vi "Merge Array.vi"(8 "Start array":i32, 9 "prev index":i32, 11 "array":T1) -> (3 "array out":T1)   [LabVIEW 2014]
uses:
  Libraries/Map Data Folder/All-Lines.ctl
  Libraries/Map Data Folder/LineCluster.ctl
  Libraries/Map Data Folder/LineConnection.ctl
  Libraries/Map Data Folder/Map Data.lvlib
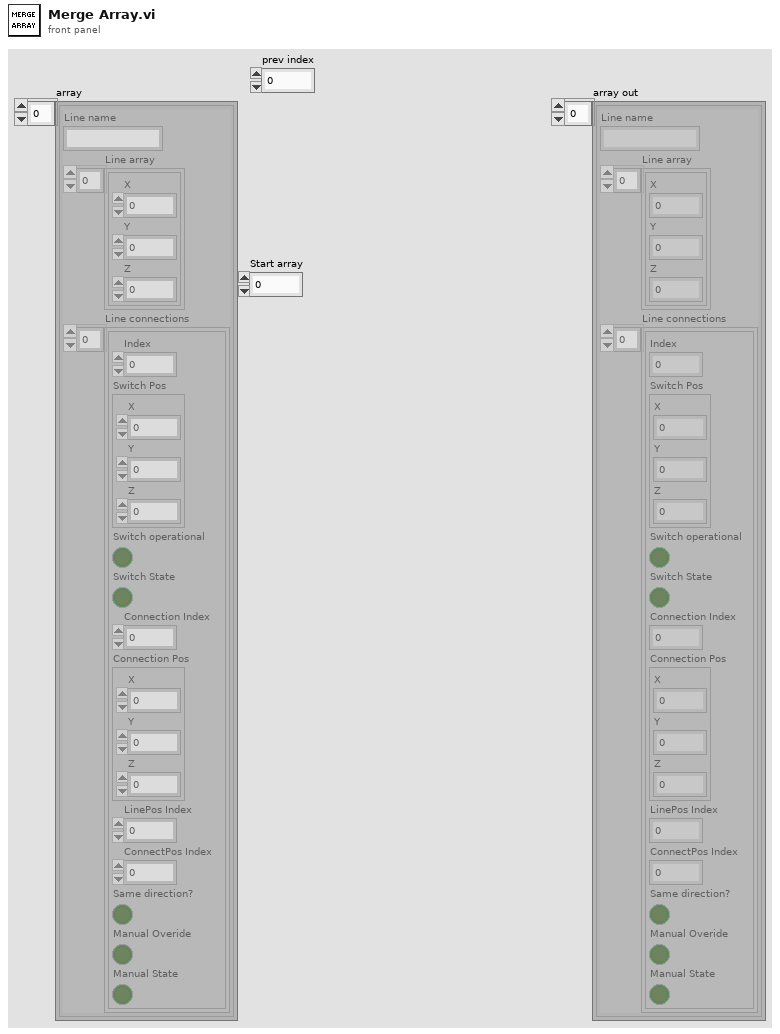
[diagram p1: front panel]
types:
  T1 = typedef "Map Data.lvlib/All-Lines.ctl" = T2[]
  T2 = typedef "Map Data.lvlib/LineCluster.ctl" = cluster{"Line name":string, "Line array":cluster{"X":dbl, "Y":dbl, "Z":dbl}[], "Line connections":T3[]}
  T3 = typedef "Map Data.lvlib/LineConnection.ctl" = cluster{"Index":i32, "Switch Pos":cluster{"X":dbl, "Y":dbl, "Z":dbl}, "Switch operational":bool, "Switch State":bool, "Connection Index":i32, "Connection Pos":cluster{"X":dbl, "Y":dbl, "Z":dbl}, "LinePos Index":i32, "ConnectPos Index":i32, "Same direction?":bool, "Manual Overide":bool, "Manual State":bool}
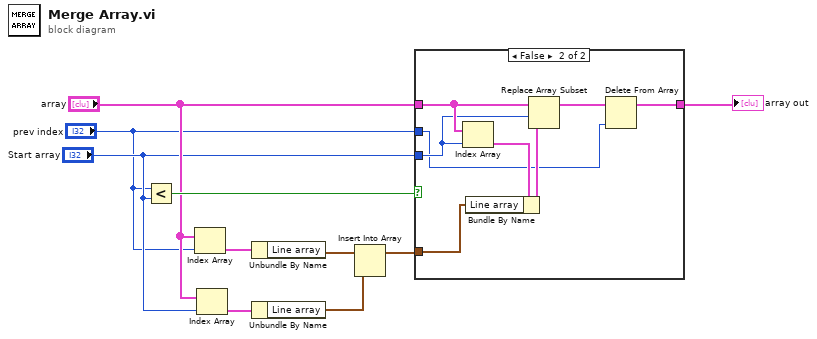
[diagram p0: block diagram]
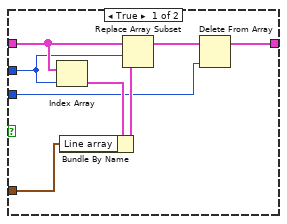
[diagram p2: hidden frame]
diagram:
  n1 = Less?(x="prev index", y="Start array") -> (x < y?=w6:bool)
  n2 = Index Array(array="array", index="prev index") -> (element=w9:T2)
  n3 = Index Array(array="array", index="Start array") -> (element=w10:T2)
  n4 = Unbundle By Name(w9) -> ("Line array"=w8:cluster{"X":dbl, "Y":dbl, "Z":dbl}[])
  n5 = Unbundle By Name(w10) -> ("Line array"=w7:cluster{"X":dbl, "Y":dbl, "Z":dbl}[])
  n6 = Insert Into Array(array=w8, new element=w7) -> (w4:cluster{"X":dbl, "Y":dbl, "Z":dbl}[])  [unwired: 1 in]
  n7 = case shown="False" w6 {
    tunnel: "array" -> [w16 w24]
    tunnel: [w12 w21] -> w1
    tunnel: w4 -> [w17 w25]
    tunnel: "Start array" -> [w11 w20]
    tunnel: "prev index" -> [w14 w19]
    frame True {
      n8 = Index Array(array=w16, index=w14) -> (element=w18:T2)
      n9 = Bundle By Name(cluster=w18, "Line array"=w17) -> (w15:T2)
      n10 = Replace Array Subset(array=w16, new element=w15, index=w14) -> (w13:T1)
      n11 = Delete From Array(array=w13, index=w11) -> (array with subset deleted=w12:T1)  [unwired: 1 in, 1 out]
    }
    frame False {
      n12 = Index Array(array=w24, index=w20) -> (element=w26:T2)
      n13 = Bundle By Name(cluster=w26, "Line array"=w25) -> (w23:T2)
      n14 = Replace Array Subset(array=w24, new element=w23, index=w20) -> (w22:T1)
      n15 = Delete From Array(array=w22, index=w19) -> (array with subset deleted=w21:T1)  [unwired: 1 in, 1 out]
    }
  }
  "array out" <- w1
